vi "usb2000Aquire.vi"(8 "error in (no error)":errorcluster, 10 "NumberOfAcquisitions (1)":i32=1, 11 "VISA resource name":refnum<visa-resource-name>) -> (0 "error out":errorcluster, 1 "MaxValue":dbl, 2 "Spectrum by Pixels":dbl[](array[numeric]), 3 "VISA resource name out":refnum<visa-resource-name>, 4 "oversaturated":bool)   [LabVIEW 2015]
uses:
  <instrlib>/Ocean Optics 2000 4000/Ocean Optics 2000 4000.lvlib
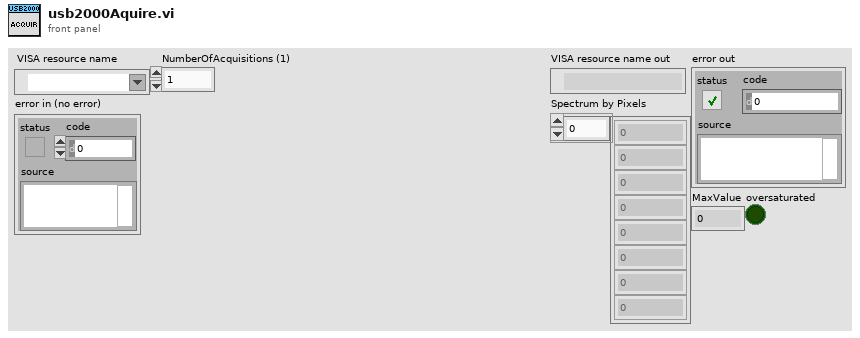
[diagram p1: front panel]
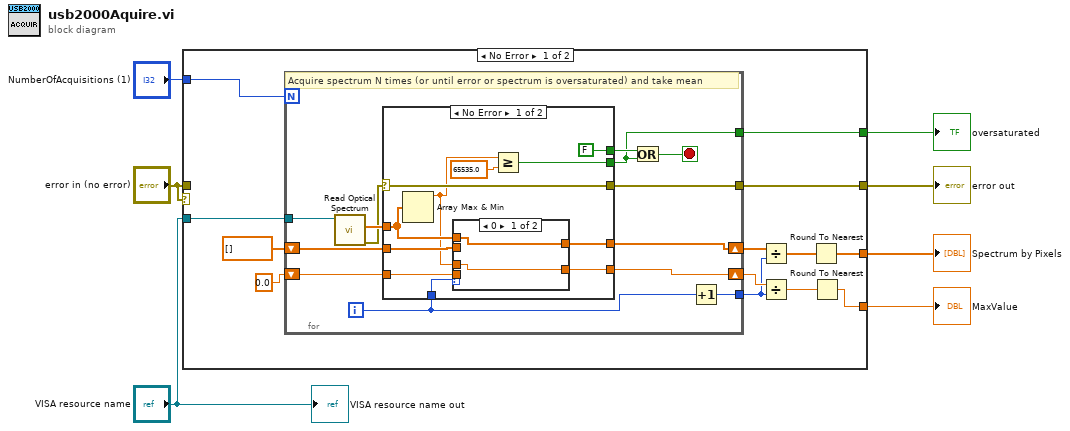
[diagram p0: block diagram]
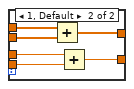
[diagram p2: hidden frame]
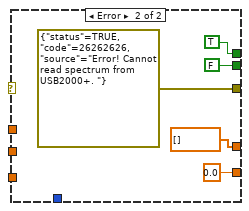
[diagram p3: hidden frame]
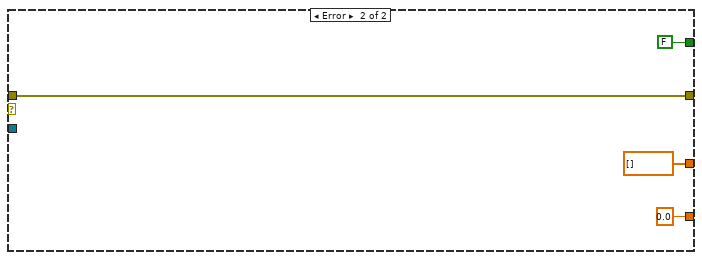
[diagram p4: hidden frame]
diagram:
  n1 = case shown="No Error" "error in (no error)" {
    tunnel: "VISA resource name" -> [w20 _]
    tunnel: "error in (no error)" -> [_ w61]
    tunnel: [w9 dbl[] [] ("Spectrum by Pixels")] -> w7
    tunnel: [w19 w61] -> w6
    tunnel: [w11 0.0] -> w5
    tunnel: [w18 FALSE] -> w4
    tunnel: "NumberOfAcquisitions (1)" -> [w17 _]
    frame No Error {
      n2 = for {
        N: w17 -> [_]
        tunnel: [w30] -> w19
        tunnel: [w27] -> w18
        tunnel: w20 -> [w33]
        shift-right: [w24] -> w14
        shift-left: dbl[] [] ("Spectrum by Pixels") -> [w25]
        shift-right: [w22] -> w13
        shift-left: 0.0 -> [w23]
        tunnel: [w29] -> w12
        i -> [w21]
        stop <- w26 stop-if-true
        # "Acquire spectrum N times (or until error or spectrum is oversaturated) and take mean"
        n3 = call <instrlib>:"Read Optical Spectrum.vi"("VISA resource name"=w33) -> ("error out"=w31:errorcluster, "Spectrum by Pixels"=w32:dbl[])  [unwired: 7 in, 2 out]
        n4 = case shown="No Error" w31 {
          selector: w31 -> [w44 _]
          tunnel: w32 -> [w39 _]
          tunnel: [w44 errorcluster {"status"=TRUE, "code"=26262626, "source"="Error! Cannot read spectrum from USB2000+. "} ("error constant")] -> w30
          tunnel: [w42 FALSE] -> w27
          tunnel: [FALSE TRUE] -> w28
          tunnel: w25 -> [w40 _]
          tunnel: [w38 dbl[] [] ("Spectrum by Pixels")] -> w24
          tunnel: w23 -> [w37 _]
          tunnel: [w35 0.0] -> w22
          tunnel: w21 -> [w34 _]
          frame No Error {
            n5 = Array Max & Min(array=w39) -> (max value=w36:dbl)  [unwired: 3 out]
            n6 = case shown="0" w34 {
              tunnel: w40 -> [_ w52]
              tunnel: w39 -> [w46 w51]
              tunnel: [w46 w50] -> w38
              tunnel: w37 -> [_ w49]
              tunnel: w36 -> [w45 w48]
              tunnel: [w45 w47] -> w35
              frame 0 {
              }
              frame 1, Default {
                n7 = Add(x=w51, y=w52) -> (x+y=w50:dbl[])
                n8 = Add(x=w48, y=w49) -> (x+y=w47:dbl)
              }
            }
            n9 = Greater Or Equal?(x=w36, y=65535.0) -> (x >= y?=w42:bool)
          }
          frame Error {
          }
        }
        n10 = Or(x=w28, y=w27) -> (x .or. y?=w26:bool)
        n11 = Increment(x=w21) -> (x+1=w29:i32)
      }
      n12 = Divide(x=w14, y=w12) -> (x/y=w10:dbl[])
      n13 = Divide(x=w13, y=w12) -> (x/y=w8:dbl)
      n14 = Round To Nearest(number=w10) -> (nearest integer value=w9:dbl[])
      n15 = Round To Nearest(number=w8) -> (nearest integer value=w11:dbl)
    }
    frame Error {
    }
  }
  "Spectrum by Pixels" <- w7
  "error out" <- w6
  "MaxValue" <- w5
  "oversaturated" <- w4
  "VISA resource name out" <- "VISA resource name"
